vi "Check Target.vi"(1 "Is 1 LBCB":bool, 2 "Other Targets":T1[](array[typedef]), 3 "Target":T1, 4 "Index":i32) -> (0 "Problems":bool)   [LabVIEW 2013]
uses:
  MixedMode/Messages/Target.ctl
  Data Access Objects/Metadata/LBCB Number.ctl
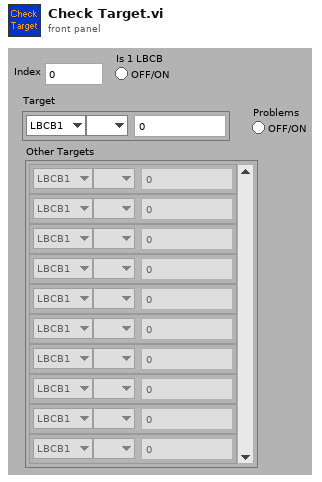
[diagram p1: front panel]
types:
  T1 = typedef "Target.ctl" = cluster{"LBCB Number":T2, "DOF Vectors":enum16{" ", "Dx", "Dy", "Dz", "Rx", "Ry", "Rz", "Fx", "Fy", "Fz", "Mx", "My", "Mz"}, "Amount":dbl}
  T2 = typedef "LBCB Number.ctl" = enum16{"LBCB1", "LBCB2"}
  T3 = enum16{" ", "Dx", "Dy", "Dz", "Rx", "Ry", "Rz", "Fx", "Fy", "Fz", "Mx", "My", "Mz"}
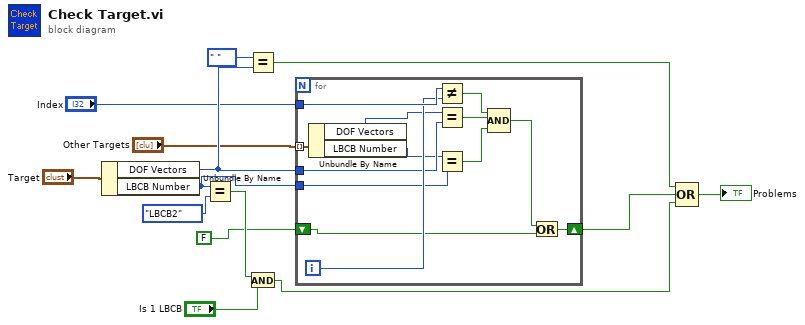
[diagram p0: block diagram]
diagram:
  n1 = Unbundle By Name("Target") -> ("DOF Vectors"=w10:T3, "LBCB Number"=w5:T2)
  n2 = Equal?(x=w5, y=LBCB_Number."LBCB2") -> (x = y?=w13:bool)
  n3 = Equal?(x=T3." ", y=w10) -> (x = y?=w7:bool)
  n4 = And(x=w13, y="Is 1 LBCB") -> (x .and. y?=w6:bool)
  n5 = for {
    tunnel: w10 -> [w23]
    tunnel: w5 -> [w21]
    shift-right: [w17] -> w2
    shift-left: FALSE ("Is 1 LBCB") -> [w15]
    tunnel: "Other Targets" -> [w27] mode=indexing
    tunnel: "Index" -> [w26]
    i -> [w25]
    n6 = Unbundle By Name(w27) -> ("DOF Vectors"=w24:T3, "LBCB Number"=w22:T2)
    n7 = Not Equal?(x=w26, y=w25) -> (x != y?=w20:bool)
    n8 = Equal?(x=w24, y=w23) -> (x = y?=w19:bool)
    n9 = Equal?(x=w22, y=w21) -> (x = y?=w18:bool)
    n10 = Compound Arithmetic op=AND(w20, w19, w18) -> (w16:bool)
    n11 = Or(x=w16, y=w15) -> (x .or. y?=w17:bool)
  }
  n12 = Compound Arithmetic op=OR(w7, w2, w6) -> (→"Problems":bool)
